vi "FPGA cRIOMain_v7.vi"() -> ()   [LabVIEW 2019]
doc: "256pt-MA"
uses:
  TypeDefs/AO mode TabCtrl.ctl
  TypeDefs/SamplingModeEnum.ctl
  TypeDefs/AI_channelEnum.ctl
  <vilib>/rvi/Emulation/niFpgaGetClockAttributes.vi
  <vilib>/rvi/Emulation/niFpgaSctlEmulationGetInTimedLoop.vi
  <vilib>/rvi/Emulation/niFpgaEmulationReportErrorSimple.vi
  <vilib>/rvi/eio/common/nirviEmuTemplateMethod_errors.vi
  <vilib>/rvi/Emulation/niFpgaEmulationIsFPGAContextNoSignature.vi
  <vilib>/rvi/DataTransferAndStorage/Container/Common/niFpgaContainerGetUniqueNameForEmu.vi
  <vilib>/rvi/Memory/Memory_Emulation/niFpgaMemoryEmulationCacheClearOnFirstRun.vi
  <vilib>/rvi/Memory/Memory_Emulation/nirvimemoryEmulationManagerCache_MakeExclusive.vi
  <vilib>/rvi/Memory/Memory_Emulation/niFpgaMemoryEmulationValidateCache.vi
  <vilib>/rvi/Memory/Memory_Emulation/nirvimemoryEmulationManagerCache_InsertValue.vi
  <vilib>/Utility/error.llb/Clear Errors.vi
  <vilib>/rvi/Memory/Memory_Emulation/nirvimemoryEmulationManagerCache_ReleaseExclusive.vi
  <vilib>/rvi/Memory/Memory_Emulation/nirvimemoryEmulationManagerCache_GetValue.vi
  <vilib>/rvi/Memory/Memory_Emulation/nirvimemoryEmulationManagerCache_SetValue.vi
  <vilib>/rvi/Emulation/niFpgaProcessEmulError.vi
  <vilib>/rvi/Emulation/niFpgaCriticalErrorInLSC.vi
  <vilib>/rvi/errors/niFpgaSetErrorForExecOnDevCompSimple.vi
  <vilib>/rvi/eio/common/nirviEmuReportErrorAndStop.vi
  <vilib>/rvi/FIFO/Fifo_Resource/nirvififoEmulationSetSize.vi
  <vilib>/rvi/FIFO/Fifo_Resource/nirviFifoEmulationQueueMgr.vi
  <instcachedir>/0/nirviFifoEmulationQueueMgr_E5CAEC123FF24DC58D834DCA3CDAA9B5.lvgen/nirviFifoEmulationQueueMgr_E5CAEC123FF24DC58D834DCA3CDAA9B5_006.vi
  <vilib>/rvi/FIFO/Fifo_Resource/nirvififoEmulationCreateLock.vi
  <vilib>/rvi/FIFO/Fifo_Resource/nirvififoEmulationObtainLock.vi
  <vilib>/rvi/FIFO/Fifo_Resource/nirvififoEmulationReleaseLock.vi
  <vilib>/rvi/occurrence/nirviWaitOnOccurrenceBase.vi
  <vilib>/rvi/errors/nirviReportUnexpectedCaseInternalError.vi
  <vilib>/rvi/errors/nirviReportUnexpectedCaseInternalError (U32).vi
  <vilib>/rvi/FIFO/Fifo_Resource/nirvififoEmulationDetermineInputValidOut.vi
  <vilib>/eio/EIONode/EIONode.xnode
  <vilib>/rvi/DataTransferAndStorage/Container/XNode/niFpgaContainer.xnode
  <vilib>/rvi/DataTransferAndStorage/Register/Emulation/niFpgaRegisterEmulation.vi
  <vilib>/rvi/FIFO/Fifo_Resource/nirvififoEmulationRead.vi
  <vilib>/rvi/FXPMathLib/FxpMul/XNode/nifxpmath_Multiplier.xnode
  <vilib>/rvi/FIFO/Fifo_Resource/nirvififoEmulationWrite.vi
  FPGA functions/FPGA functions.lvlib
  <vilib>/rvi/FXPMathLib/sim/FxpSim.dll
panel:
  out "AI Processing\nLoop Rate to high?":bool
  in  "AI Process Time [ticks]":u32=125
  in  "Select Channel":T1
  out "Unable to\nsample at desired\nSample Rate?":bool
  out "Processing Loop time [ticks]":u32
  in  "Sampling Mode":T2
  in  "AO mode":T3
  in  "AO Out [V]":fxp<+/-,18,5> format="%#.6g"
  in  "AO enable?":bool
  out "AI In [V]":fxp<+/-,28,5> format="%#.6g"
  out "FPGA AO DMA\nOverflow?":bool
  out "Int. Output":fxp<+/-,20,5> format="%.17g"
  out "Raw AI Input":fxp<+/-,28,5> format="%.21g"
  in  "Sample Time [ticks]":u32=125
  out "AO Loop time [ticks]":u32
  out "AI Loop time [ticks]":u32
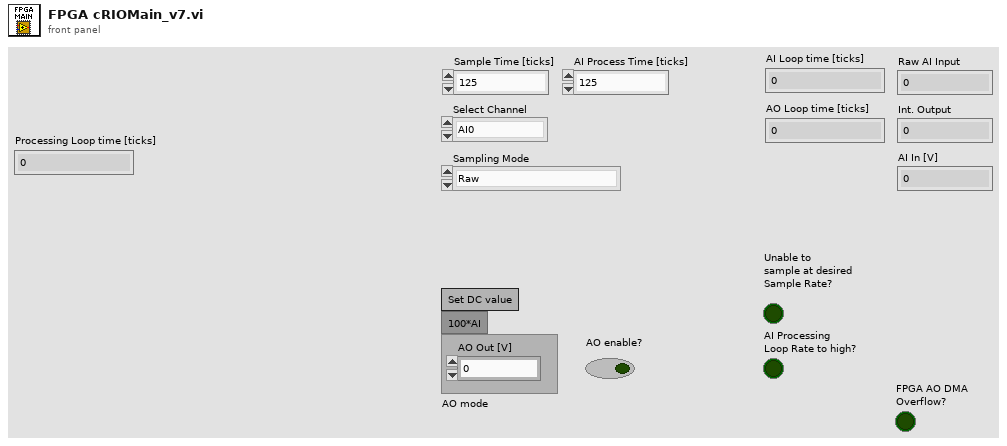
[diagram p1: front panel]
types:
  T1 = typedef "AI_channelEnum.ctl" = enum16{"AI0", "AI1", "AI2", "AI3"}
  T2 = typedef "SamplingModeEnum.ctl" = enum16{"Raw", "M64 (ReSpl)", "M128 (ReSpl)", "M256 (ReSpl)", "MA (AI)", "4pt MA (AI) + M64 (ReSpl)", "LPF (Proc.)", "4pt MA (AI) + LPF (Proc.)", "4pt MA (Proc.) + LPF (Proc.)"}
  T3 = typedef "AO mode TabCtrl.ctl" = enum32{"Set DC value", "100*AI"}
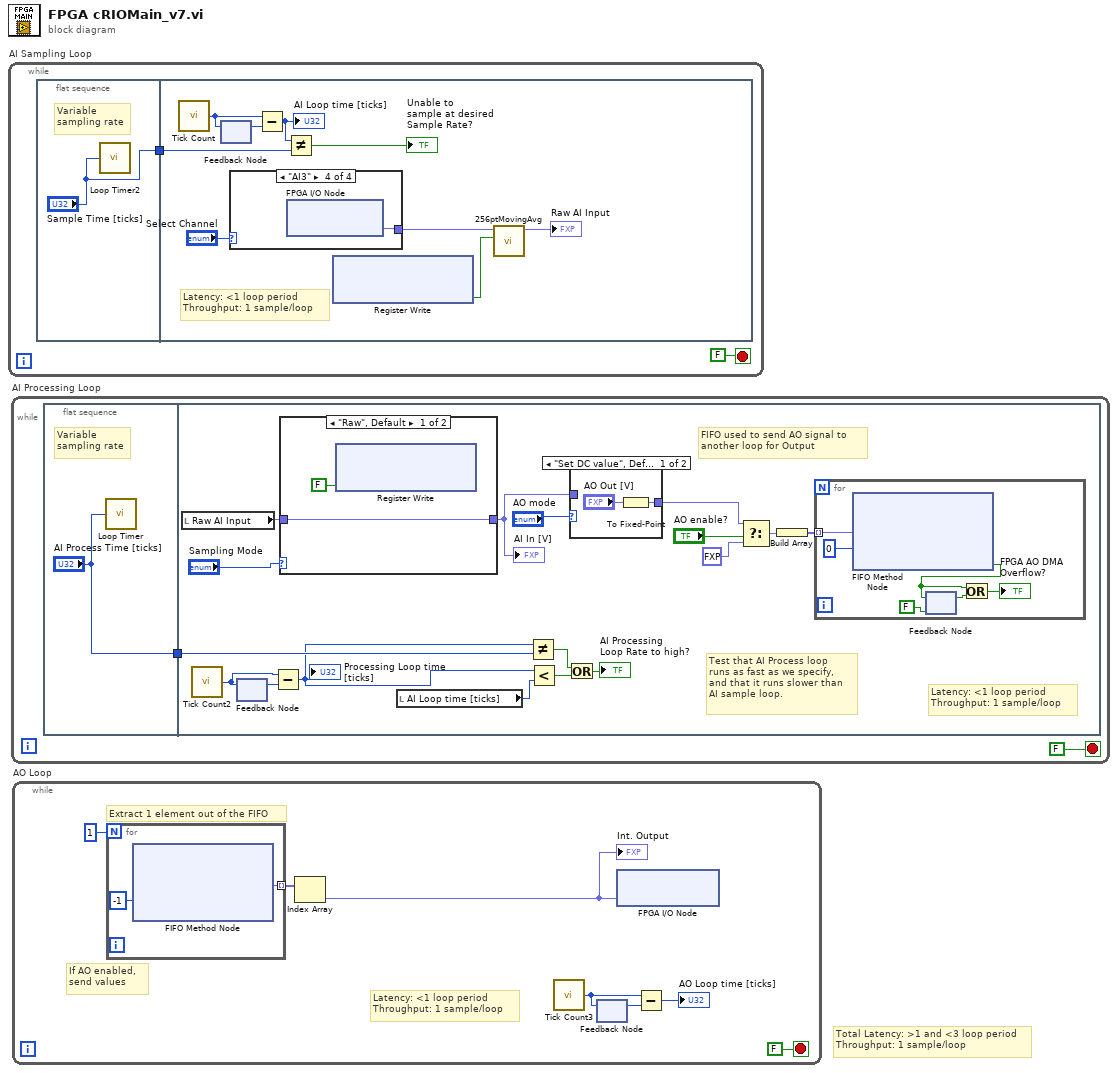
[diagram p0: block diagram]
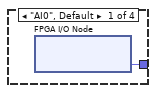
[diagram p2: hidden frame]
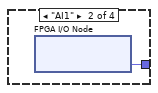
[diagram p3: hidden frame]
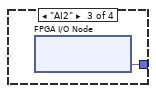
[diagram p4: hidden frame]
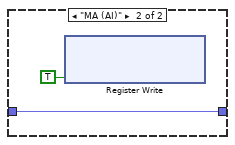
[diagram p5: hidden frame]
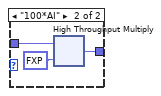
[diagram p6: hidden frame]
diagram:
  # "Total Latency: >1 and <3 loop period\nThroughput: 1 sample/loop"
  n1 = while "AI Sampling Loop" {
    stop <- FALSE stop-if-true
    n2 = flat-sequence {
      tunnel: ["Sample Time [ticks]"] -> w1
      tunnel: w1 -> [w9]
      frame #0 {
        # "Variable\nsampling rate"
        n3 = call "Loop Timer2"("Count(Ticks)"="Sample Time [ticks]") -> ()  [unwired: 1 out]
      }
      frame #1 {
        # "Latency: <1 loop period\nThroughput: 1 sample/loop"
        n4 = call "Tick Count"() -> ("Tick Count(Ticks)"=w12:u32)
        n5 = feedback #1() -> (w11:u32)  [unwired: 1 in]
        n6 = feedback-in #1(w12) -> ()
        n7 = case shown="\"AI3\"" "Select Channel" {
          tunnel: [w13 w14 w15 w16] -> w6
          frame "AI0", Default {
            n8 = xnode "FPGA I/O Node"() -> ("Mod4/AI0"=w13:fxp<+/-,24,5>)  [unwired: 1 in, 1 out]
          }
          frame "AI1" {
            n9 = xnode "FPGA I/O Node"() -> ("Mod4/AI1"=w14:fxp<+/-,24,5>)  [unwired: 1 in, 1 out]
          }
          frame "AI2" {
            n10 = xnode "FPGA I/O Node"() -> ("Mod4/AI2"=w15:fxp<+/-,24,5>)  [unwired: 1 in, 1 out]
          }
          frame "AI3" {
            n11 = xnode "FPGA I/O Node"() -> ("Mod4/AI3"=w16:fxp<+/-,24,5>)  [unwired: 1 in, 1 out]
          }
        }
        n12 = Subtract(x=w12, y=w11) -> (x-y=w10:u32)
        "AI Loop time [ticks]" <- w10
        n13 = Not Equal?(x=w10, y=w9) -> (x != y?=→"Unable to\nsample at desired\nSample Rate?":bool)
        n14 = xnode ("Register Write")() -> ("Data"=w5:bool)  [unwired: 1 in, 1 out]
        n15 = call "256ptMovingAvg.vi"("Enable?"=w5, "Raw input"=w6) -> ("Output"=→"Raw AI Input":fxp<+/-,28,5>)  [unwired: 9 in]
      }
    }
  }
  n16 = while "AI Processing Loop" {
    stop <- FALSE stop-if-true
    n17 = flat-sequence {
      tunnel: ["AI Process Time [ticks]"] -> w17
      tunnel: w17 -> [w21]
      frame #0 {
        # "Variable\nsampling rate"
        n18 = call "Loop Timer"("Count(Ticks)"="AI Process Time [ticks]") -> ()  [unwired: 1 out]
      }
      frame #1 {
        # "Test that AI Process loop\nruns as fast as we specify,\nand that it runs slower than \nAI sample loop."
        # "Latency: <1 loop period\nThroughput: 1 sample/loop"
        # "FIFO used to send AO signal to \nanother loop for Output"
        n19 = local read "Raw AI Input"() -> (w25:fxp<+/-,28,5>)
        n20 = call "Tick Count2"() -> ("Tick Count(Ticks)"=w35:u32)
        n21 = feedback #2() -> (w36:u32)  [unwired: 1 in]
        n22 = feedback-in #2(w35) -> ()
        n23 = Subtract(x=w35, y=w36) -> (x-y=w20:u32)
        "Processing Loop time [ticks]" <- w20
        n24 = case shown="\"Raw\", Default" "Sampling Mode" {
          tunnel: [w37 w39] -> w33
          tunnel: w25 -> [w37 w39]
          frame "Raw", Default {
            n25 = xnode ("Register Write")("Data"=FALSE) -> ()  [unwired: 1 in, 1 out]
          }
          frame "MA (AI)" {
            n26 = xnode ("Register Write")("Data"=TRUE) -> ()  [unwired: 1 in, 1 out]
          }
        }
        "AI In [V]" <- w33
        n27 = local read "AI Loop time [ticks]"() -> (w26:u32)
        n28 = Not Equal?(x=w20, y=w21) -> (x != y?=w23:bool)
        n29 = Less?(x=w20, y=w26) -> (x < y?=w22:bool)
        n30 = Or(x=w23, y=w22) -> (x .or. y?=→"AI Processing\nLoop Rate to high?":bool)
        n31 = case shown="\"Set DC value\", Default" "AO mode" {
          tunnel: [w42 w43] -> w30
          tunnel: w33 -> [_ w45]
          frame "Set DC value", Default {
            n32 = To Fixed-Point(number="AO Out [V]") -> (fixed-point=w42:fxp<+/-,20,5>)  [unwired: 1 in]
          }
          frame "100*AI" {
            n33 = xnode ("High Throughput Multiply")("x"=w45, "y"=fxp<+,5,7> 100.0) -> ("x*y"=w43:fxp<+/-,20,5>)
          }
        }
        n34 = Select(t=w30, s="AO enable?", f=fxp<+/-,20,5> 0.0) -> (s? t:f=w34:fxp<+/-,20,5>)
        n35 = Build Array(w34) -> (w29:fxp<+/-,20,5>[])
        n36 = for {
          tunnel: w29 -> [w46] mode=indexing
          n37 = xnode ("FIFO Method Node")("Element"=w46, "Timeout"=0) -> ("Timed Out?"=w47:bool)  [unwired: 1 in, 1 out]
          n38 = feedback-in #3(w47) -> ()
          n39 = feedback #3(FALSE ("Timed Out?")) -> (w50:bool)
          n40 = Or(x=w47, y=w50) -> (x .or. y?=→"FPGA AO DMA\nOverflow?":bool)
        }
      }
    }
  }
  n41 = while "AO Loop" {
    stop <- FALSE stop-if-true
    # "Latency: <1 loop period\nThroughput: 1 sample/loop"
    # "If AO enabled, \nsend values"
    # "Extract 1 element out of the FIFO"
    n42 = for {
      N: 1 -> [_]
      tunnel: [w60] -> w54 mode=indexing
      n43 = xnode ("FIFO Method Node")("Timeout"=-1) -> ("Element"=w60:fxp<+/-,20,5>)  [unwired: 1 in, 2 out]
    }
    n44 = Index Array(array=w54) -> (element=w52:fxp<+/-,20,5>)  [unwired: 1 in]
    "Int. Output" <- w52
    n45 = call "Tick Count3"() -> ("Tick Count(Ticks)"=w57:u32)
    n46 = feedback #4() -> (w56:u32)  [unwired: 1 in]
    n47 = feedback-in #4(w57) -> ()
    n48 = xnode "FPGA I/O Node"("Mod3/AO1"=w52) -> ()  [unwired: 1 in, 1 out]
    n49 = Subtract(x=w57, y=w56) -> (x-y=→"AO Loop time [ticks]":u32)
  }
